vi "Invalid Version Format--error.vi"() -> (0 "error out":errorcluster)   [LabVIEW 2025]
doc: "Indicates that the specified Version has an invalid format."
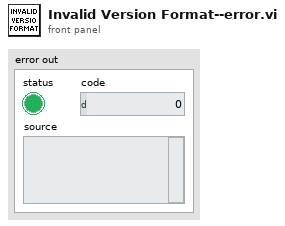
[diagram p1: front panel]
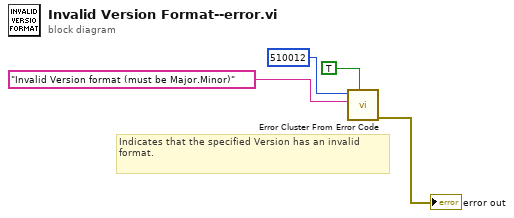
[diagram p0: block diagram]
diagram:
  # "Indicates that the specified Version has an invalid format."
  n1 = call <vilib>:"Error Cluster From Error Code.vi"("show call chain? (False)"=TRUE, "error message (\"\")"="Invalid Version format (must be Major.Minor)" ("error message (\"\")"), "error code (0)"=510012) -> ("error out"=→"error out":errorcluster)  [unwired: 6 in]
